vi "GermanInfo_Check_chosen_field (SubVI).vi"(8 "Error In":errorcluster, 11 "Settings in":T2 {"Permanent data"."Окно с настройками"."Образец" items=["1", "2", "3"]; "Permanent data"."Окно с настройками"."Условия окружающей среды" items=["Нормальная температура", "Максимальная температура", "Минимальная температура", "Вибрации типа А", "Вибрации типа Б"]; "Permanent data"."Окно с настройками"."Напряжение источника" items=["12", "24"]; "Permanent data"."Окно с настройками"."Режим звонка" items=["Автоматически (AT)", "Автоматически (реле)", "Вручную"]}) -> (0 "Error Out":errorcluster, 3 "Settings out":T2 {"Permanent data"."Окно с настройками"."Образец" items=["1", "2", "3"]; "Permanent data"."Окно с настройками"."Условия окружающей среды" items=["Нормальная температура", "Максимальная температура", "Минимальная температура", "Вибрации типа А", "Вибрации типа Б"]; "Permanent data"."Окно с настройками"."Напряжение источника" items=["12", "24"]; "Permanent data"."Окно с настройками"."Режим звонка" items=["Автоматически (AT)", "Автоматически (реле)", "Вручную"]})   [LabVIEW 2018]
uses:
  CSMinfo.ctl
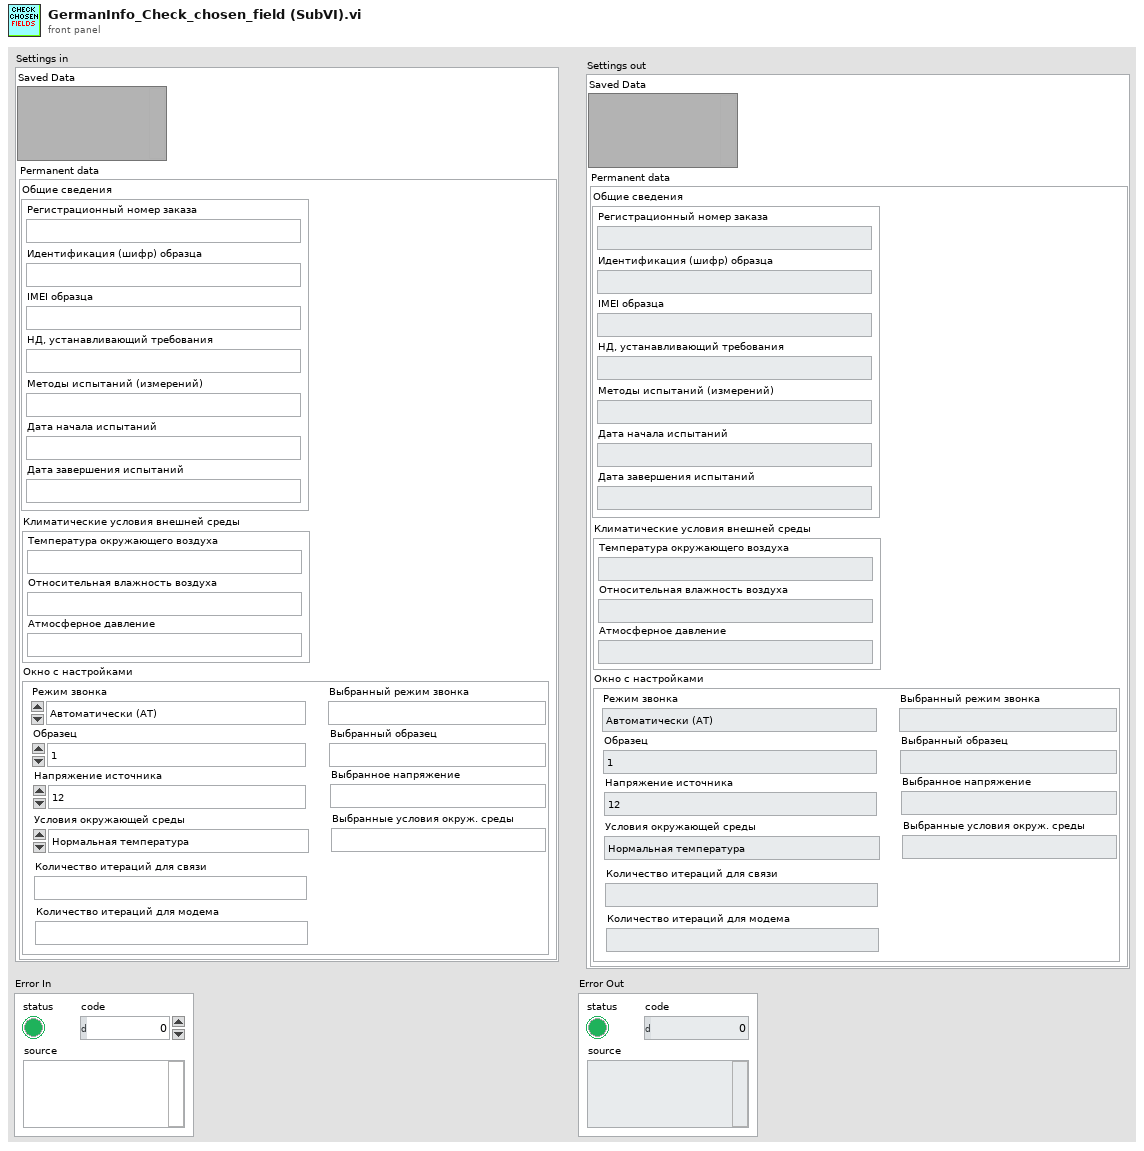
[diagram p1: front panel]
types:
  T1 = typedef "CSMinfo.ctl" = cluster{"Общие сведения":cluster{"Регистрационный номер заказа":string, "Идентификация (шифр) образца":string, "IMEI образца":string, "НД, устанавливающий требования":string, "Методы испытаний (измерений)":string, "Дата начала испытаний":string, "Дата завершения испытаний":string}, "Климатические условия внешней среды":cluster{"Температура окружающего воздуха":string, "Относительная влажность воздуха":string, "Атмосферное давление":string}, "Окно с настройками":cluster{"Режим звонка":u16, "Напряжение источника":u16, "Условия окружающей среды":u16, "Образец":u16, "Количество итераций для модема":string, "Количество итераций для связи":string, "Выбранный режим звонка":string, "Выбранный образец":string, "Выбранное напряжение":string, "Выбранные условия окруж. среды":string}}
  T2 = cluster{"Saved Data":variant, "Permanent data":T1}
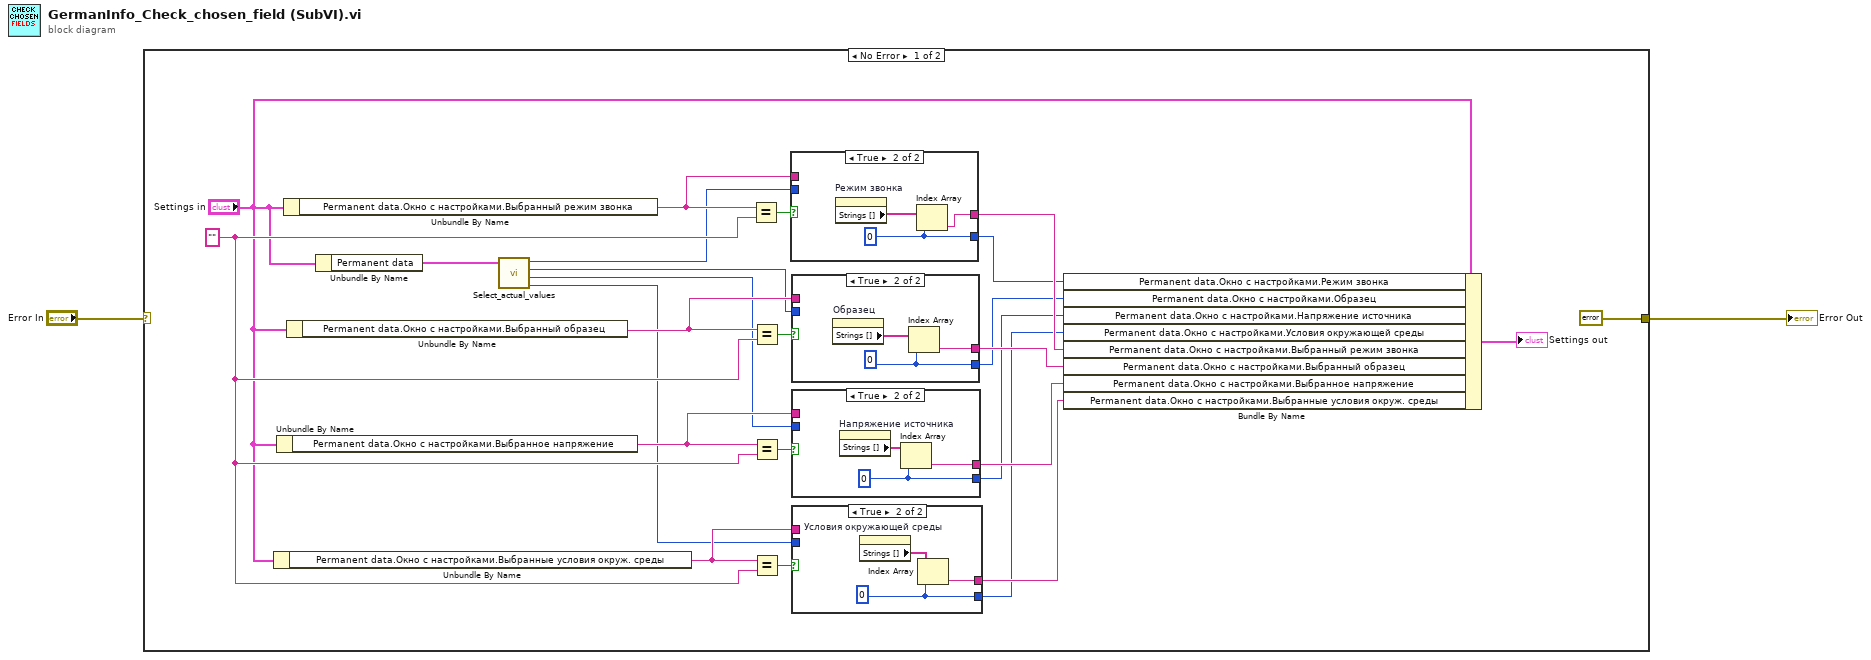
[diagram p0: block diagram]
diagram:
  n1 = case shown="No Error" "Error In" {
    selector: "Error In" -> [_ w48]
    tunnel: [errorcluster {"status"=FALSE, "code"=0, "source"=""} ("error IO") w48] -> w1
    frame No Error {
      w19 = "" ("replace string (\"\")")
      n2 = Unbundle By Name("Settings in") -> ("Permanent data.Окно с настройками.Выбранные условия окруж. среды"=w21:string)
      n3 = Unbundle By Name("Settings in") -> ("Permanent data.Окно с настройками.Выбранное напряжение"=w22:string)
      n4 = Unbundle By Name("Settings in") -> ("Permanent data.Окно с настройками.Выбранный режим звонка"=w23:string)
      n5 = Unbundle By Name("Settings in") -> ("Permanent data.Окно с настройками.Выбранный образец"=w24:string)
      n6 = Unbundle By Name("Settings in") -> ("Permanent data"=w7:T1)
      n7 = call "Select_actual_values.vi"("CSMinfo in"=w7) -> ("Условия окружающей среды"=w3:u16, "Напряжение источника"=w4:u16, "Образец"=w5:u16, "Режим звонка"=w6:u16)  [unwired: 7 in]
      n8 = Equal?(x=w23, y=w19) -> (x = y?=w27:bool)
      n9 = Equal?(x=w24, y=w19) -> (x = y?=w26:bool)
      n10 = Equal?(x=w22, y=w19) -> (x = y?=w25:bool)
      n11 = Equal?(x=w21, y=w19) -> (x = y?=w20:bool)
      n12 = case shown="True" w27 {
        tunnel: [w44 w46] -> w18
        tunnel: w23 -> [w44 _]
        tunnel: [w43 w45] -> w9
        tunnel: w6 -> [w43 _]
        frame False {
        }
        frame True {
          w45 = 0 ("index")
          n13 = property on="Режим звонка" class="Ring (strict)"() -> ("Strings []"=w47:string[])  [unwired: 2 in, 2 out]
          n14 = Index Array(array=w47, index=w45) -> (element=w46:string)
        }
      }
      n15 = case shown="True" w26 {
        tunnel: [w39 w41] -> w17
        tunnel: w24 -> [w39 _]
        tunnel: [w38 w40] -> w10
        tunnel: w5 -> [w38 _]
        frame False {
        }
        frame True {
          w40 = 0 ("index")
          n16 = property on="Образец" class="Ring (strict)"() -> ("Strings []"=w42:string[])  [unwired: 2 in, 2 out]
          n17 = Index Array(array=w42, index=w40) -> (element=w41:string)
        }
      }
      n18 = case shown="True" w25 {
        tunnel: [w34 w36] -> w16
        tunnel: w22 -> [w34 _]
        tunnel: [w33 w35] -> w11
        tunnel: w4 -> [w33 _]
        frame False {
        }
        frame True {
          w35 = 0 ("index")
          n19 = property on="Напряжение источника" class="Ring (strict)"() -> ("Strings []"=w37:string[])  [unwired: 2 in, 2 out]
          n20 = Index Array(array=w37, index=w35) -> (element=w36:string)
        }
      }
      n21 = case shown="True" w20 {
        tunnel: [w29 w31] -> w15
        tunnel: w21 -> [w29 _]
        tunnel: [w28 w30] -> w12
        tunnel: w3 -> [w28 _]
        frame False {
        }
        frame True {
          w30 = 0 ("index")
          n22 = property on="Условия окружающей среды" class="Ring (strict)"() -> ("Strings []"=w32:string[])  [unwired: 2 in, 2 out]
          n23 = Index Array(array=w32, index=w30) -> (element=w31:string)
        }
      }
      n24 = Bundle By Name(cluster="Settings in", "Permanent data.Окно с настройками.Режим звонка"=w9, "Permanent data.Окно с настройками.Образец"=w10, "Permanent data.Окно с настройками.Напряжение источника"=w11, "Permanent data.Окно с настройками.Условия окружающей среды"=w12, "Permanent data.Окно с настройками.Выбранный режим звонка"=w18, "Permanent data.Окно с настройками.Выбранный образец"=w17, "Permanent data.Окно с настройками.Выбранное напряжение"=w16, "Permanent data.Окно с настройками.Выбранные условия окруж. среды"=w15) -> (→"Settings out":T2)
    }
    frame Error {
    }
  }
  "Error Out" <- w1
